vi "Autonomous Independent.vi"() -> ()   [LabVIEW 2016]
doc: "This VI is called when autonomous begins, and will automatically be terminated when autonomous ends. You can carry out timed or sensor driven robot movement independently without needing to return to the caller."
uses:
  <vilib>/Rock Robotics/Network Tables/NT Read Number.vi
  Global 2.vi
  Systems/Global 1.vi
panel:
  out "Elapsed Time (s) 2":dbl=0.2559828758239746 caption="Elapsed Time (s)"
  out "Time has Elapsed 2":bool=TRUE caption="Time has Elapsed"
  out "Present (s) 2":dbl=3576145380.999535 caption="Present (s)"
  out "Present (s)":dbl=3576102803.059525
  out "Time has Elapsed":bool=TRUE
  out "Elapsed Time (s)":dbl=0.25415611267089844
  out "Gyro":dbl=0.5670717799999513
  in  "Oscillate effort":dbl=0.25 format="%#_13g"
  out "Auto Mode":dbl=2.0
  in  "Auton_Modes":T1(array[cluster])=[{"Actions"=[{"Effort"=0.55, "Duration"=3.5, "Action"=enum."Nothing", "Encoder"=0.0, "Condition"=FALSE}, {"Effort"=0.0, "Duration"=0.0, "Action"=enum."Nothing", "Encoder"=0.0, "Condition"=FALSE}]}, {"Actions"=[{"Effort"=0.0, "Duration"=0.1, "Action"=enum."Drive Encoder Reset", "Encoder"=0.0, "Condition"=FALSE}, {"Effort"=0.0, "Duration"=0.1, "Action"=enum."Gyro Reset", "Encoder"=0.0, "Condition"=FALSE}, {"Effort"=0.0, "Duration"=4.0, "Action"=enum."Drive", "Encoder"=62.0, "Condition"=FALSE}, {"Effort"=0.15, "Duration"=0.1, "Action"=enum."Turn", "Encoder"=-55.0, "Condition"=FALSE}, {"Effort"=0.0, "Duration"=0.1, "Action"=enum."Gyro Reset", "Encoder"=0.0, "Condition"=FALSE}, {"Effort"=0.0, "Duration"=0.1, "Action"=enum."Drive Encoder Reset", "Encoder"=0.0, "Condition"=FALSE}, {"Effort"=0.0, "Duration"=4.0, "Action"=enum."Drive", "Encoder"=76.0, "Condition"=FALSE}, {"Effort"=1.0, "Duration"=0.25, "Action"=enum."Gear0", "Encoder"=0.0, "Condition"=FALSE}, {"Effort"=0.0, "Duration"=0.1, "Action"=enum."Drive Encoder Reset", "Encoder"=3.0, "Condition"=FALSE}, {"Effort"=0.0, "Duration"=3.0, "Action"=enum."Drive", "Encoder"=-36.0, "Condition"=FALSE}, {"Effort"=0.08, "Duration"=0.0, "Action"=enum."Turn", "Encoder"=15.5, "Condition"=FALSE}, {"Effort"=0.0, "Duration"=0.1, "Action"=enum."Gyro Reset", "Encoder"=0.0, "Condition"=FALSE}, {"Effort"=0.0, "Duration"=0.5, "Action"=enum."Drive Encoder Reset", "Encoder"=0.0, "Condition"=FALSE}, {"Effort"=0.0, "Duration"=5.0, "Action"=enum."Drive", "Encoder"=-94.0, "Condition"=TRUE}]}, {"Actions"=[{"Effort"=0.0, "Duration"=0.1, "Action"=enum."Drive Encoder Reset", "Encoder"=0.0, "Condition"=FALSE}, {"Effort"=0.0, "Duration"=0.1, "Action"=enum."Gyro Reset", "Encoder"=0.0, "Condition"=FALSE}, {"Effort"=0.11, "Duration"=4.0, "Action"=enum."Drive", "Encoder"=74.0, "Condition"=FALSE}, {"Effort"=1.0, "Duration"=0.5, "Action"=enum."Gear0", "Encoder"=0.0, "Condition"=FALSE}, {"Effort"=1.0, "Duration"=0.0, "Action"=enum."Nothing", "Encoder"=0.0, "Condition"=FALSE}, {"Effort"=1.0, "Duration"=0.0, "Action"=enum."Nothing", "Encoder"=0.0, "Condition"=FALSE}, {"Effort"=0.0, "Duration"=0.0, "Action"=enum."Drive Encoder Reset", "Encoder"=0.0, "Condition"=FALSE}, {"Effort"=0.0, "Duration"=0.0, "Action"=enum."Nothing", "Encoder"=0.0, "Condition"=FALSE}, {"Effort"=0.0, "Duration"=0.0, "Action"=enum."Nothing", "Encoder"=0.0, "Condition"=FALSE}, {"Effort"=0.0, "Duration"=10000.0, "Action"=enum."Drive", "Encoder"=-24.0, "Condition"=FALSE}, {"Effort"=0.0, "Duration"=0.0, "Action"=enum."Drive Encoder Reset", "Encoder"=0.0, "Condition"=FALSE}, {"Effort"=-0.4, "Duration"=5.0, "Action"=enum."Nothing", "Encoder"=70.0, "Condition"=FALSE}]}, {"Actions"=[{"Effort"=0.0, "Duration"=0.1, "Action"=enum."Drive Encoder Reset", "Encoder"=6.462, "Condition"=FALSE}, {"Effort"=0.0, "Duration"=0.1, "Action"=enum."Gyro Reset", "Encoder"=0.0, "Condition"=FALSE}, {"Effort"=0.0, "Duration"=1.0, "Action"=enum."Drive", "Encoder"=60.0, "Condition"=FALSE}, {"Effort"=0.15, "Duration"=0.1, "Action"=enum."Turn", "Encoder"=55.0, "Condition"=FALSE}, {"Effort"=0.0, "Duration"=0.1, "Action"=enum."Gyro Reset", "Encoder"=0.0, "Condition"=FALSE}, {"Effort"=-0.25, "Duration"=0.0, "Action"=enum."Drive Encoder Reset", "Encoder"=7.5, "Condition"=FALSE}, {"Effort"=0.0, "Duration"=4.0, "Action"=enum."Drive", "Encoder"=76.0, "Condition"=FALSE}, {"Effort"=1.0, "Duration"=0.25, "Action"=enum."Gear0", "Encoder"=0.0, "Condition"=FALSE}, {"Effort"=0.0, "Duration"=0.1, "Action"=enum."Drive Encoder Reset", "Encoder"=0.0, "Condition"=FALSE}, {"Effort"=0.0, "Duration"=3.0, "Action"=enum."Drive", "Encoder"=-36.0, "Condition"=FALSE}, {"Effort"=0.08, "Duration"=0.0, "Action"=enum."Turn", "Encoder"=-60.0, "Condition"=FALSE}, {"Effort"=0.0, "Duration"=0.1, "Action"=enum."Gyro Reset", "Encoder"=0.0, "Condition"=FALSE}, {"Effort"=0.0, "Duration"=0.5, "Action"=enum."Drive Encoder Reset", "Encoder"=0.0, "Condition"=FALSE}, {"Effort"=0.0, "Duration"=5.0, "Action"=enum."Drive", "Encoder"=30.0, "Condition"=TRUE}]}, {"Actions"=[{"Effort"=0.0, "Duration"=0.1, "Action"=enum."Drive Encoder Reset", "Encoder"=6.462, "Condition"=FALSE}, {"Effort"=0.0, "Duration"=0.1, "Action"=enum."Gyro Reset", "Encoder"=0.0, "Condition"=FALSE}, {"Effort"=0.0, "Duration"=1.0, "Action"=enum."Drive", "Encoder"=60.0, "Condition"=FALSE}, {"Effort"=0.15, "Duration"=0.1, "Action"=enum."Turn", "Encoder"=-55.0, "Condition"=FALSE}, {"Effort"=0.0, "Duration"=0.1, "Action"=enum."Gyro Reset", "Encoder"=0.0, "Condition"=FALSE}, {"Effort"=-0.25, "Duration"=0.0, "Action"=enum."Drive Encoder Reset", "Encoder"=7.5, "Condition"=FALSE}, {"Effort"=0.0, "Duration"=4.0, "Action"=enum."Drive", "Encoder"=76.0, "Condition"=FALSE}, {"Effort"=1.0, "Duration"=0.25, "Action"=enum."Gear0", "Encoder"=0.0, "Condition"=FALSE}, {"Effort"=0.0, "Duration"=0.1, "Action"=enum."Drive Encoder Reset", "Encoder"=0.0, "Condition"=FALSE}, {"Effort"=0.0, "Duration"=3.0, "Action"=enum."Drive", "Encoder"=-36.0, "Condition"=FALSE}, {"Effort"=0.08, "Duration"=0.0, "Action"=enum."Turn", "Encoder"=60.0, "Condition"=FALSE}, {"Effort"=0.0, "Duration"=0.1, "Action"=enum."Gyro Reset", "Encoder"=0.0, "Condition"=FALSE}, {"Effort"=0.0, "Duration"=0.5, "Action"=enum."Drive Encoder Reset", "Encoder"=0.0, "Condition"=FALSE}, {"Effort"=0.0, "Duration"=5.0, "Action"=enum."Drive", "Encoder"=30.0, "Condition"=TRUE}]}, {"Actions"=[{"Effort"=0.0, "Duration"=0.1, "Action"=enum."Drive Encoder Reset", "Encoder"=0.0, "Condition"=FALSE}, {"Effort"=0.0, "Duration"=0.1, "Action"=enum."Gyro Reset", "Encoder"=0.0, "Condition"=FALSE}, {"Effort"=0.0, "Duration"=4.0, "Action"=enum."Drive", "Encoder"=62.0, "Condition"=FALSE}, {"Effort"=0.15, "Duration"=0.1, "Action"=enum."Turn", "Encoder"=55.0, "Condition"=FALSE}, {"Effort"=0.0, "Duration"=0.1, "Action"=enum."Gyro Reset", "Encoder"=0.0, "Condition"=FALSE}, {"Effort"=0.0, "Duration"=0.1, "Action"=enum."Drive Encoder Reset", "Encoder"=0.0, "Condition"=FALSE}, {"Effort"=0.0, "Duration"=4.0, "Action"=enum."Drive", "Encoder"=76.0, "Condition"=FALSE}, {"Effort"=1.0, "Duration"=0.25, "Action"=enum."Gear0", "Encoder"=0.0, "Condition"=FALSE}, {"Effort"=0.0, "Duration"=0.1, "Action"=enum."Drive Encoder Reset", "Encoder"=3.0, "Condition"=FALSE}, {"Effort"=0.0, "Duration"=3.0, "Action"=enum."Drive", "Encoder"=-36.0, "Condition"=FALSE}, {"Effort"=0.08, "Duration"=0.0, "Action"=enum."Turn", "Encoder"=-15.5, "Condition"=FALSE}, {"Effort"=0.0, "Duration"=0.1, "Action"=enum."Gyro Reset", "Encoder"=0.0, "Condition"=FALSE}, {"Effort"=0.0, "Duration"=0.5, "Action"=enum."Drive Encoder Reset", "Encoder"=0.0, "Condition"=FALSE}, {"Effort"=0.0, "Duration"=5.0, "Action"=enum."Drive", "Encoder"=-94.0, "Condition"=TRUE}, {"Effort"=0.0, "Duration"=10.0, "Action"=enum."Shoot", "Encoder"=0.0, "Condition"=FALSE}]}, {"Actions"=[{"Effort"=0.0, "Duration"=0.1, "Action"=enum."Drive Encoder Reset", "Encoder"=0.0, "Condition"=FALSE}, {"Effort"=0.0, "Duration"=0.1, "Action"=enum."Gyro Reset", "Encoder"=0.0, "Condition"=FALSE}, {"Effort"=0.2, "Duration"=5.0, "Action"=enum."Drive", "Encoder"=110.0, "Condition"=FALSE}, {"Effort"=0.75, "Duration"=1.0, "Action"=enum."Nothing", "Encoder"=0.0, "Condition"=FALSE}, {"Effort"=0.0, "Duration"=1.0, "Action"=enum."Nothing", "Encoder"=0.0, "Condition"=FALSE}, {"Effort"=0.0, "Duration"=0.0, "Action"=enum."Nothing", "Encoder"=0.0, "Condition"=FALSE}]}, {"Actions"=[{"Effort"=0.0, "Duration"=0.1, "Action"=enum."Drive Encoder Reset", "Encoder"=0.0, "Condition"=FALSE}, {"Effort"=0.0, "Duration"=0.1, "Action"=enum."Gyro Reset", "Encoder"=0.0, "Condition"=FALSE}, {"Effort"=0.3, "Duration"=0.0, "Action"=enum."Drive", "Encoder"=24.0, "Condition"=FALSE}, {"Effort"=0.3, "Duration"=3.0, "Action"=enum."Nothing", "Encoder"=0.0, "Condition"=FALSE}, {"Effort"=0.3, "Duration"=2.0, "Action"=enum."Vision Correction", "Encoder"=30.0, "Condition"=FALSE}, {"Effort"=0.2, "Duration"=1.0, "Action"=enum."Drive", "Encoder"=18.5, "Condition"=TRUE}, {"Effort"=1.0, "Duration"=0.0, "Action"=enum."Gear0", "Encoder"=0.0, "Condition"=FALSE}, {"Effort"=-0.2, "Duration"=1.3, "Action"=enum."Drive", "Encoder"=30.0, "Condition"=TRUE}, {"Effort"=0.0, "Duration"=3.0, "Action"=enum."Nothing", "Encoder"=0.0, "Condition"=FALSE}, {"Effort"=0.03, "Duration"=0.0, "Action"=enum."Turn", "Encoder"=0.0, "Condition"=FALSE}, {"Effort"=0.0, "Duration"=0.0, "Action"=enum."Drive", "Encoder"=0.0, "Condition"=FALSE}]}, {"Actions"=[{"Effort"=0.0, "Duration"=0.0, "Action"=enum."Nothing", "Encoder"=0.0, "Condition"=FALSE}]}, {"Actions"=[{"Effort"=0.0, "Duration"=2.5, "Action"=enum."Shoot", "Encoder"=0.0, "Condition"=FALSE}, {"Effort"=0.0, "Duration"=5.0, "Action"=enum."Index", "Encoder"=0.0, "Condition"=FALSE}, {"Effort"=0.25, "Duration"=3.5, "Action"=enum."Nothing", "Encoder"=88.0, "Condition"=FALSE}, {"Effort"=1.0, "Duration"=1.0, "Action"=enum."Nothing", "Encoder"=0.0, "Condition"=FALSE}, {"Effort"=1.0, "Duration"=1.0, "Action"=enum."Nothing", "Encoder"=0.0, "Condition"=FALSE}, {"Effort"=1.0, "Duration"=0.5, "Action"=enum."Nothing", "Encoder"=0.0, "Condition"=FALSE}, {"Effort"=0.0, "Duration"=0.0, "Action"=enum."Nothing", "Encoder"=0.0, "Condition"=FALSE}, {"Effort"=-0.25, "Duration"=0.0, "Action"=enum."Nothing", "Encoder"=3.0, "Condition"=FALSE}, {"Effort"=0.0, "Duration"=0.0, "Action"=enum."Nothing", "Encoder"=0.0, "Condition"=FALSE}, {"Effort"=0.25, "Duration"=0.0, "Action"=enum."Nothing", "Encoder"=24.0, "Condition"=FALSE}, {"Effort"=0.0, "Duration"=0.0, "Action"=enum."Nothing", "Encoder"=0.0, "Condition"=FALSE}, {"Effort"=-0.25, "Duration"=0.0, "Action"=enum."Nothing", "Encoder"=12.0, "Condition"=FALSE}]}, {"Actions"=[{"Effort"=0.0, "Duration"=0.1, "Action"=enum."Drive Encoder Reset", "Encoder"=0.0, "Condition"=FALSE}, {"Effort"=0.0, "Duration"=1.0, "Action"=enum."Gyro Reset", "Encoder"=0.0, "Condition"=FALSE}, {"Effort"=0.3, "Duration"=1.4, "Action"=enum."Drive", "Encoder"=88.0, "Condition"=FALSE}, {"Effort"=0.3, "Duration"=3.0, "Action"=enum."Turn", "Encoder"=2.0, "Condition"=FALSE}, {"Effort"=1.0, "Duration"=1.0, "Action"=enum."Nothing", "Encoder"=0.0, "Condition"=FALSE}, {"Effort"=1.0, "Duration"=1.0, "Action"=enum."Nothing", "Encoder"=0.0, "Condition"=FALSE}, {"Effort"=0.0, "Duration"=0.0, "Action"=enum."Nothing", "Encoder"=0.0, "Condition"=FALSE}, {"Effort"=-0.25, "Duration"=0.0, "Action"=enum."Nothing", "Encoder"=3.0, "Condition"=FALSE}, {"Effort"=0.0, "Duration"=0.0, "Action"=enum."Nothing", "Encoder"=0.0, "Condition"=FALSE}, {"Effort"=0.25, "Duration"=0.0, "Action"=enum."Nothing", "Encoder"=24.0, "Condition"=FALSE}, {"Effort"=0.0, "Duration"=0.0, "Action"=enum."Nothing", "Encoder"=0.0, "Condition"=FALSE}, {"Effort"=-0.25, "Duration"=0.0, "Action"=enum."Nothing", "Encoder"=12.0, "Condition"=FALSE}]}, {"Actions"=[{"Effort"=0.0, "Duration"=1.0, "Action"=enum."Drive Encoder Reset", "Encoder"=0.0, "Condition"=FALSE}, {"Effort"=0.0, "Duration"=1.0, "Action"=enum."Shoot", "Encoder"=0.0, "Condition"=FALSE}, {"Effort"=0.25, "Duration"=5.0, "Action"=enum."Index", "Encoder"=88.0, "Condition"=FALSE}, {"Effort"=1.0, "Duration"=1.0, "Action"=enum."Nothing", "Encoder"=0.0, "Condition"=FALSE}, {"Effort"=1.0, "Duration"=1.0, "Action"=enum."Nothing", "Encoder"=0.0, "Condition"=FALSE}, {"Effort"=1.0, "Duration"=0.5, "Action"=enum."Nothing", "Encoder"=0.0, "Condition"=FALSE}, {"Effort"=0.0, "Duration"=0.0, "Action"=enum."Nothing", "Encoder"=0.0, "Condition"=FALSE}, {"Effort"=-0.25, "Duration"=0.0, "Action"=enum."Nothing", "Encoder"=3.0, "Condition"=FALSE}, {"Effort"=0.0, "Duration"=0.0, "Action"=enum."Nothing", "Encoder"=0.0, "Condition"=FALSE}, {"Effort"=0.25, "Duration"=0.0, "Action"=enum."Nothing", "Encoder"=24.0, "Condition"=FALSE}, {"Effort"=0.0, "Duration"=0.0, "Action"=enum."Nothing", "Encoder"=0.0, "Condition"=FALSE}, {"Effort"=-0.25, "Duration"=0.0, "Action"=enum."Nothing", "Encoder"=12.0, "Condition"=FALSE}]}, {"Actions"=[{"Effort"=0.0, "Duration"=0.1, "Action"=enum."Drive Encoder Reset", "Encoder"=0.0, "Condition"=FALSE}, {"Effort"=0.0, "Duration"=1.0, "Action"=enum."Gyro Reset", "Encoder"=0.0, "Condition"=FALSE}, {"Effort"=0.0, "Duration"=20.0, "Action"=enum."Drive", "Encoder"=60.0, "Condition"=FALSE}, {"Effort"=0.3, "Duration"=4.0, "Action"=enum."Nothing", "Encoder"=0.0, "Condition"=FALSE}, {"Effort"=1.0, "Duration"=1.0, "Action"=enum."Nothing", "Encoder"=0.0, "Condition"=FALSE}, {"Effort"=1.0, "Duration"=0.5, "Action"=enum."Nothing", "Encoder"=0.0, "Condition"=FALSE}, {"Effort"=0.0, "Duration"=0.0, "Action"=enum."Nothing", "Encoder"=0.0, "Condition"=FALSE}, {"Effort"=0.3, "Duration"=0.5, "Action"=enum."Nothing", "Encoder"=24.0, "Condition"=TRUE}, {"Effort"=0.0, "Duration"=0.0, "Action"=enum."Nothing", "Encoder"=0.0, "Condition"=FALSE}, {"Effort"=-0.2, "Duration"=2.0, "Action"=enum."Nothing", "Encoder"=24.0, "Condition"=TRUE}, {"Effort"=0.0, "Duration"=0.0, "Action"=enum."Nothing", "Encoder"=0.0, "Condition"=FALSE}, {"Effort"=-0.25, "Duration"=0.0, "Action"=enum."Nothing", "Encoder"=12.0, "Condition"=FALSE}]}, {"Actions"=[{"Effort"=0.0, "Duration"=0.1, "Action"=enum."Drive Encoder Reset", "Encoder"=0.0, "Condition"=FALSE}, {"Effort"=0.0, "Duration"=0.1, "Action"=enum."Gyro Reset", "Encoder"=0.0, "Condition"=FALSE}, {"Effort"=0.0, "Duration"=4.0, "Action"=enum."Nothing", "Encoder"=4.0, "Condition"=FALSE}, {"Effort"=0.3, "Duration"=0.1, "Action"=enum."Vision Correction", "Encoder"=24.0, "Condition"=FALSE}, {"Effort"=0.0, "Duration"=0.1, "Action"=enum."Nothing", "Encoder"=0.0, "Condition"=FALSE}, {"Effort"=0.3, "Duration"=4.0, "Action"=enum."Nothing", "Encoder"=68.17, "Condition"=FALSE}, {"Effort"=1.0, "Duration"=0.25, "Action"=enum."Nothing", "Encoder"=0.0, "Condition"=FALSE}, {"Effort"=0.0, "Duration"=0.0, "Action"=enum."Nothing", "Encoder"=3.0, "Condition"=FALSE}, {"Effort"=-0.3, "Duration"=3.0, "Action"=enum."Nothing", "Encoder"=36.0, "Condition"=FALSE}, {"Effort"=0.15, "Duration"=0.0, "Action"=enum."Nothing", "Encoder"=31.5, "Condition"=FALSE}, {"Effort"=0.0, "Duration"=0.1, "Action"=enum."Nothing", "Encoder"=0.0, "Condition"=FALSE}]}]
  # "Nothing"
  # "Boiler Right Right side gear"
  # "Middle Gear"
  # "Boiler Right Left Side Gear"
  # "Boiler Left RightSide Gear"
  # "Boiler Left Left Side Gear"
  # "Drive"
  # "Vision Correction"
  # "Hopper"
  # "10 ball"
  # "Farside"
  # "Boilerside-10 ball"
  # "Auto 5"
  # "Auto 6"
  # "Auto 6"
  # "Auto 7"
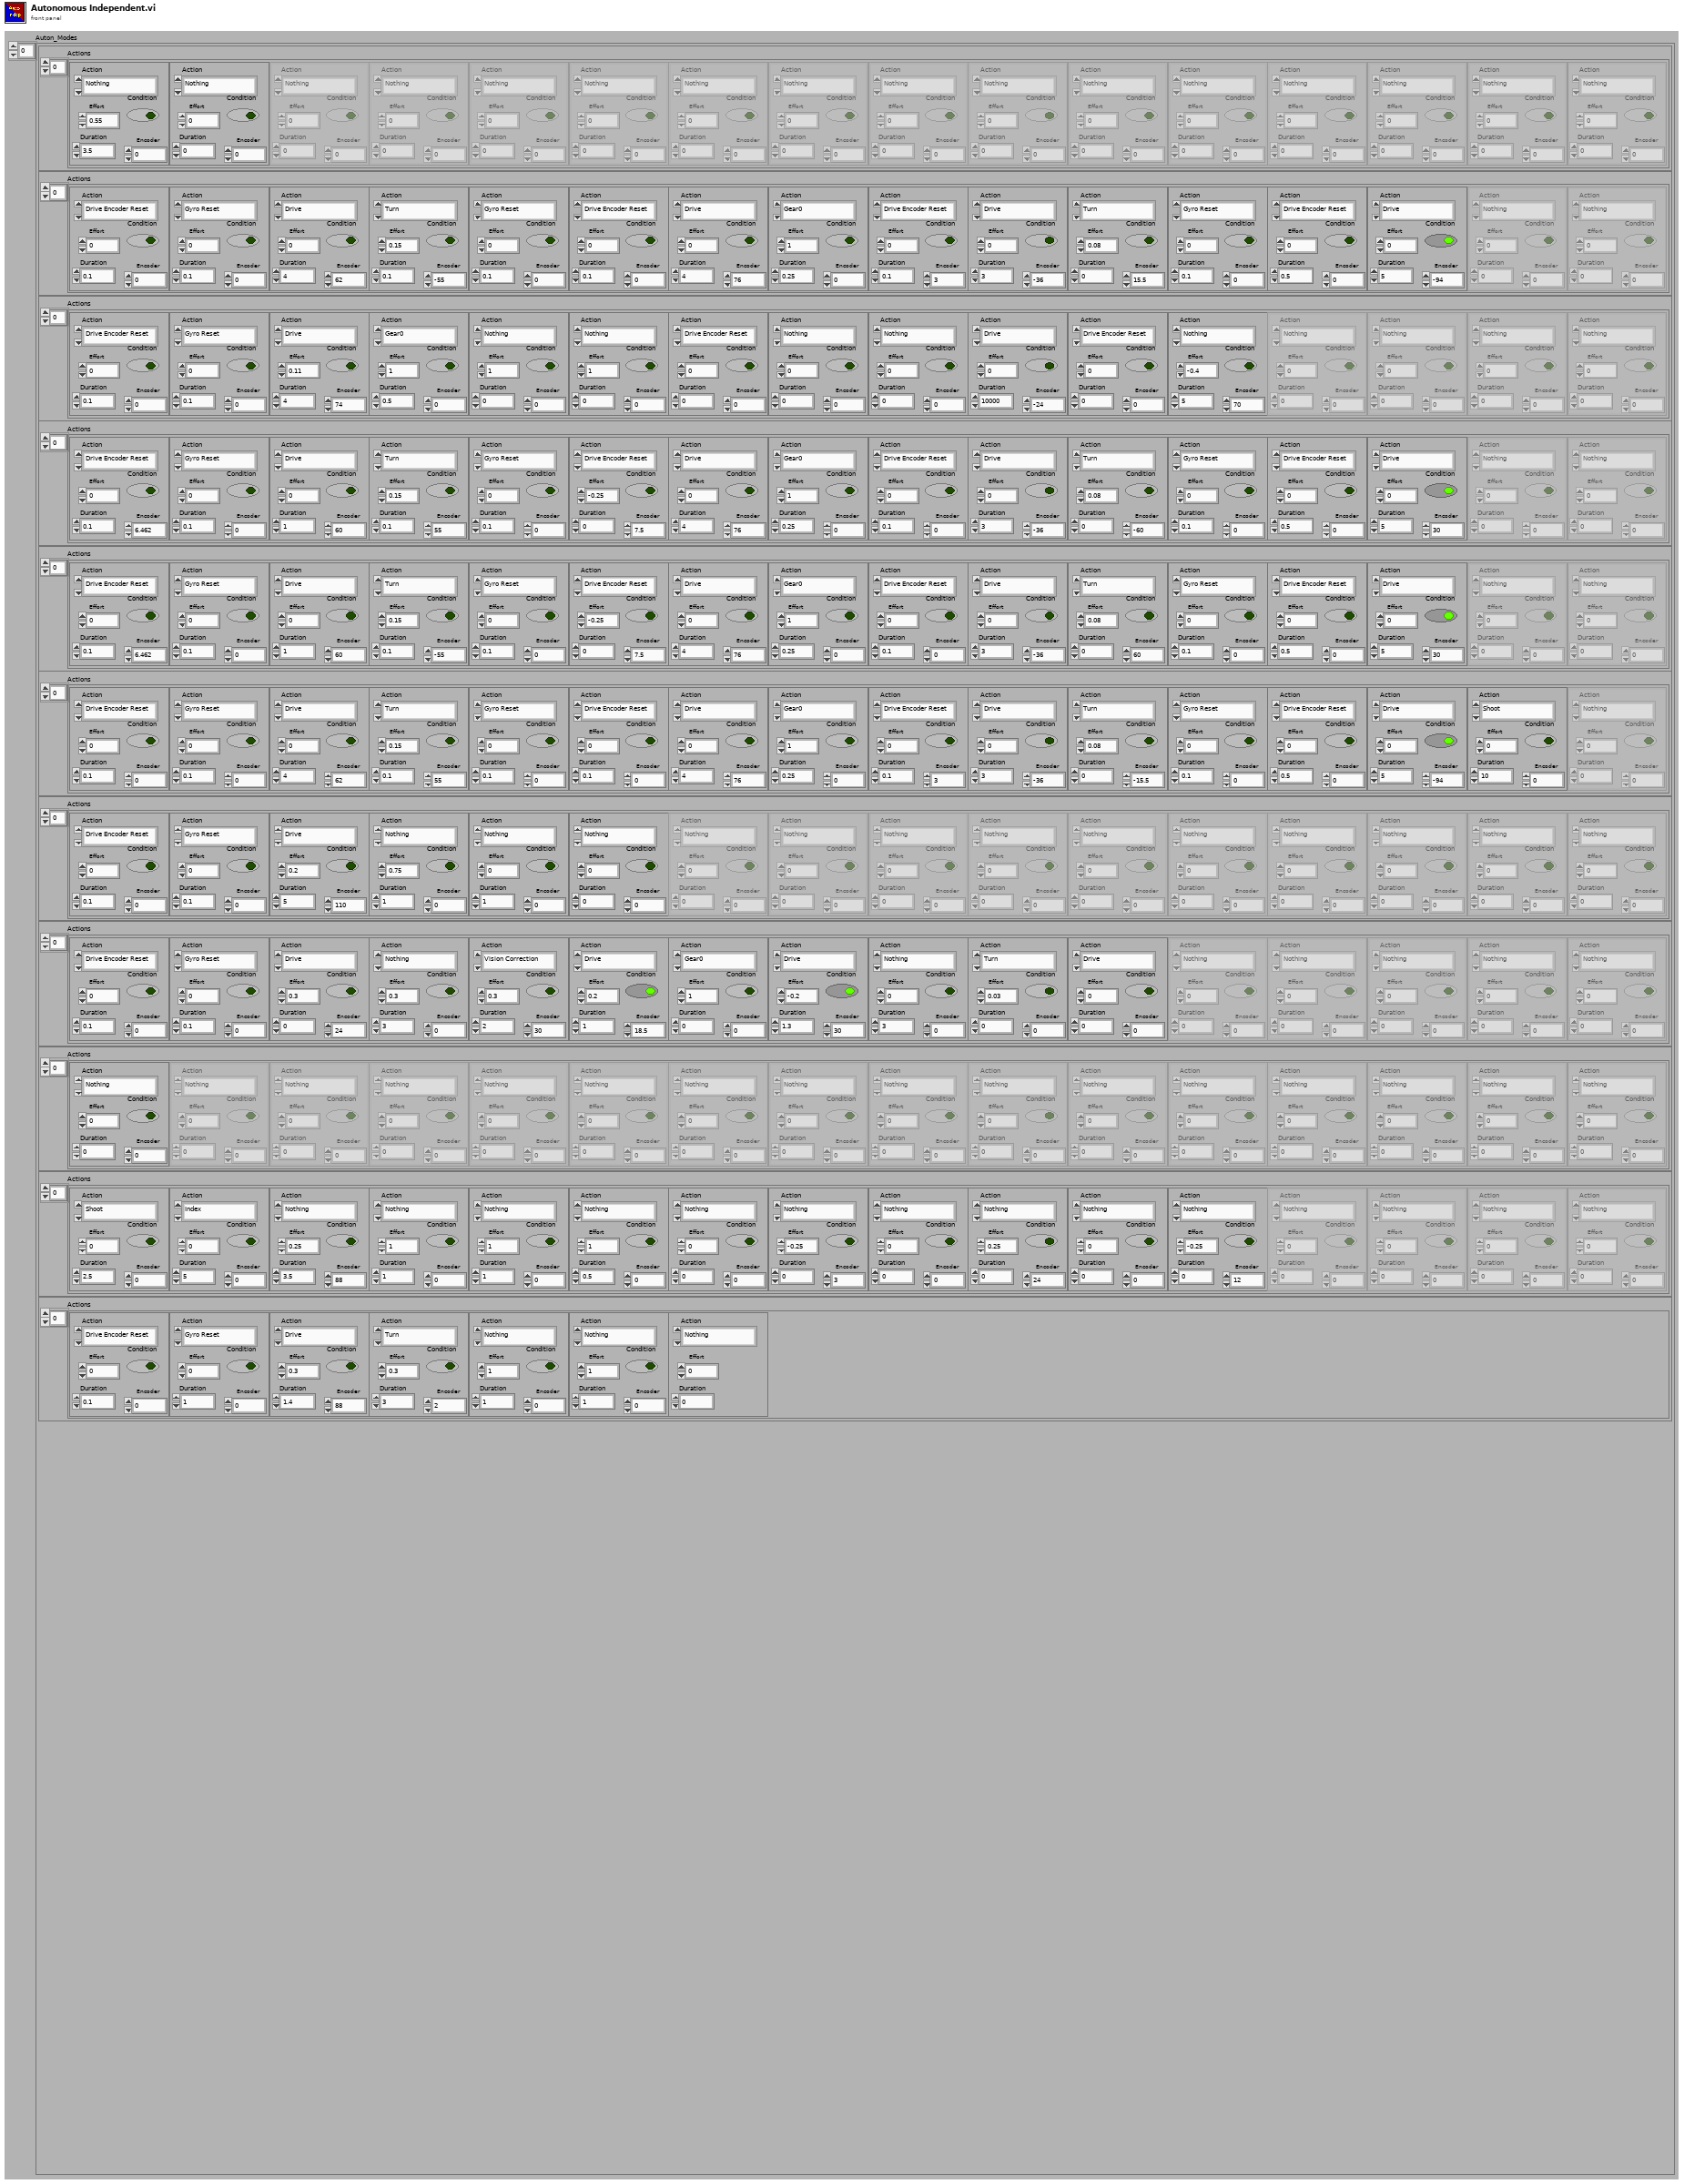
[diagram p1: front panel]
types:
  T1 = cluster{"Actions":cluster{"Effort":dbl, "Duration":dbl, "Action":enum16{"Nothing", "Drive", "Vision Correction", "Turn", "Gear0", "Gear1", "Climb", "Intake", "Index", "Shoot", "Test", "Drive Encoder Reset", "Gyro Reset"}, "Encoder":dbl, "Condition":bool}[]}[]
  T2 = cluster{"Actions":cluster{"Effort":dbl, "Duration":dbl, "Action":enum16{"Nothing", "Drive", "Vision Correction", "Turn", "Gear0", "Gear1", "Climb", "Intake", "Index", "Shoot", "Test", "Drive Encoder Reset", "Gyro Reset"}, "Encoder":dbl, "Condition":bool}[]}
  T3 = cluster{"Effort":dbl, "Duration":dbl, "Action":enum16{"Nothing", "Drive", "Vision Correction", "Turn", "Gear0", "Gear1", "Climb", "Intake", "Index", "Shoot", "Test", "Drive Encoder Reset", "Gyro Reset"}, "Encoder":dbl, "Condition":bool}[]
  T4 = enum16{"Nothing", "Drive", "Vision Correction", "Turn", "Gear0", "Gear1", "Climb", "Intake", "Index", "Shoot", "Test", "Drive Encoder Reset", "Gyro Reset"}
  T5 = typedef "WPI_MotorControlDeviceRef.ctl" = cluster{"DeviceStatus":errorcluster, "Type":T6, "PWM":cluster{"PWM Channel":T7, "DeadBand":T8}, "CAN":cluster{"Device Number":u8, "SetOutput VI Ref":variant, "GetOutput VI Ref":variant, "Enable VI Ref":variant, "Disable VI Ref":variant, "Data":variant}, "Invert":bool}
  T6 = typedef "WPI_MotorControlType.ctl" = enum16{"PWM", "CAN"}
  T7 = typedef "FPGA_DIOPWMChannel.ctl" = enum8{"PWM 0", "PWM 1", "PWM 2", "PWM 3", "PWM 4", "PWM 5", "PWM 6", "PWM 7", "PWM 8", "PWM 9", "PWM MXP 0", "PWM MXP 1", "PWM MXP 2", "PWM MXP 3", "PWM MXP 4", "PWM MXP 5", "PWM MXP 6", "PWM MXP 7", "PWM MXP 8", "PWM MXP 9", "Invalid"}
  T8 = typedef "WPI_PWMDeadband.ctl" = cluster{"Name":string, "maxPositivePwm":i32, "minPositivePwm":i32, "centerPwm":i32, "maxNegativePwm":i32, "minNegativePwm":i32, "angularRange":u16}
  T9 = typedef "WPI_CANTalonSRX_GlobalStatus.ctl" = cluster{"Applied Throttle":dbl, "Module Enabled":bool, "CAN Error":errorcluster, "Closed Loop Error":dbl, "Forward Limit Switch Closed":bool, "Reverse Limit Switch Closed":bool, "Sensor Position":dbl, "Sensor Velocity":dbl, "Current":dbl, "Sticky Fault - Over Temp":bool, "Sticky Fault - Under Voltage":bool, "Sticky Fault - Forward Limit":bool, "Sticky Fault - Reverse Limit":bool, "Sticky Fault - Forward Soft Limit":bool, "Sticky Fault - Reverse Soft Limit":bool, "Brake is Enabled":bool, "Encoder Position":dbl, "Encoder Velocity":dbl, "Encoder Index Count":dbl, "Encoder A Pin State":bool, "Encoder B Pin State":bool, "Encoder Index Pin State":bool, "Analog In":dbl, "Analog In Velocity":dbl, "Temperature (C)":dbl, "Battery Voltage":dbl, "Control 5 Is Supported":bool, "Current Profile Slot Select":dbl, "Pos Div 8":bool, "Vel Div 4":bool, "Pulse Width Position":i32, "Pulse Width Velocity":i32, "Pulse Width Rise To Rise (us)":i32, "Pulse Width Rise To Fall (us)":i32, "Mot Prof Active Is Under Run":bool, "Mot Prof Active Has Under Run":bool, "Mot Prof Active Is Last":bool, "Mot Prof Active Velocity Only":bool, "Mot Prof Active Is Valid":bool, "Mot Prof Buffer Is Full":bool, "Mot Prof Active Profile Slot Select":i32, "Mot Prof NextID":i32, "Mot Prof Count":i32, "Mot Prof Active Velocity":dbl, "Mot Prof Active Position":dbl, "Mot Prof Output Enable":i32}
  T10 = typedef "WPI_GyroDevRef.ctl" = cluster{"DevStatus":errorcluster, "Analog Channel":T11, "Offset":dbl, "Gain (VoltsPerDegree/Second)":dbl, "Gyro Type":enum16{"Analog", "XRS450"}, "Handle":i32, "SPI Bus":T12, "Device Found":bool, "Sample Rate":dbl, "Calibrate On Open":bool}
  T11 = typedef "FPGA_AIChannel.ctl" = enum8{"AI 0", "AI 1", "AI 2", "AI 3", "AI MXP 0", "AI MXP 1", "AI MXP 2", "AI MXP 3", "Invalid"}
  T12 = typedef "spi_bus.ctl" = enum16{"SPI On-Board, CS0", "SPI On-Board, CS1", "SPI On-Board, CS2", "SPI On-Board, CS3", "SPI MXP", "Invalid"}
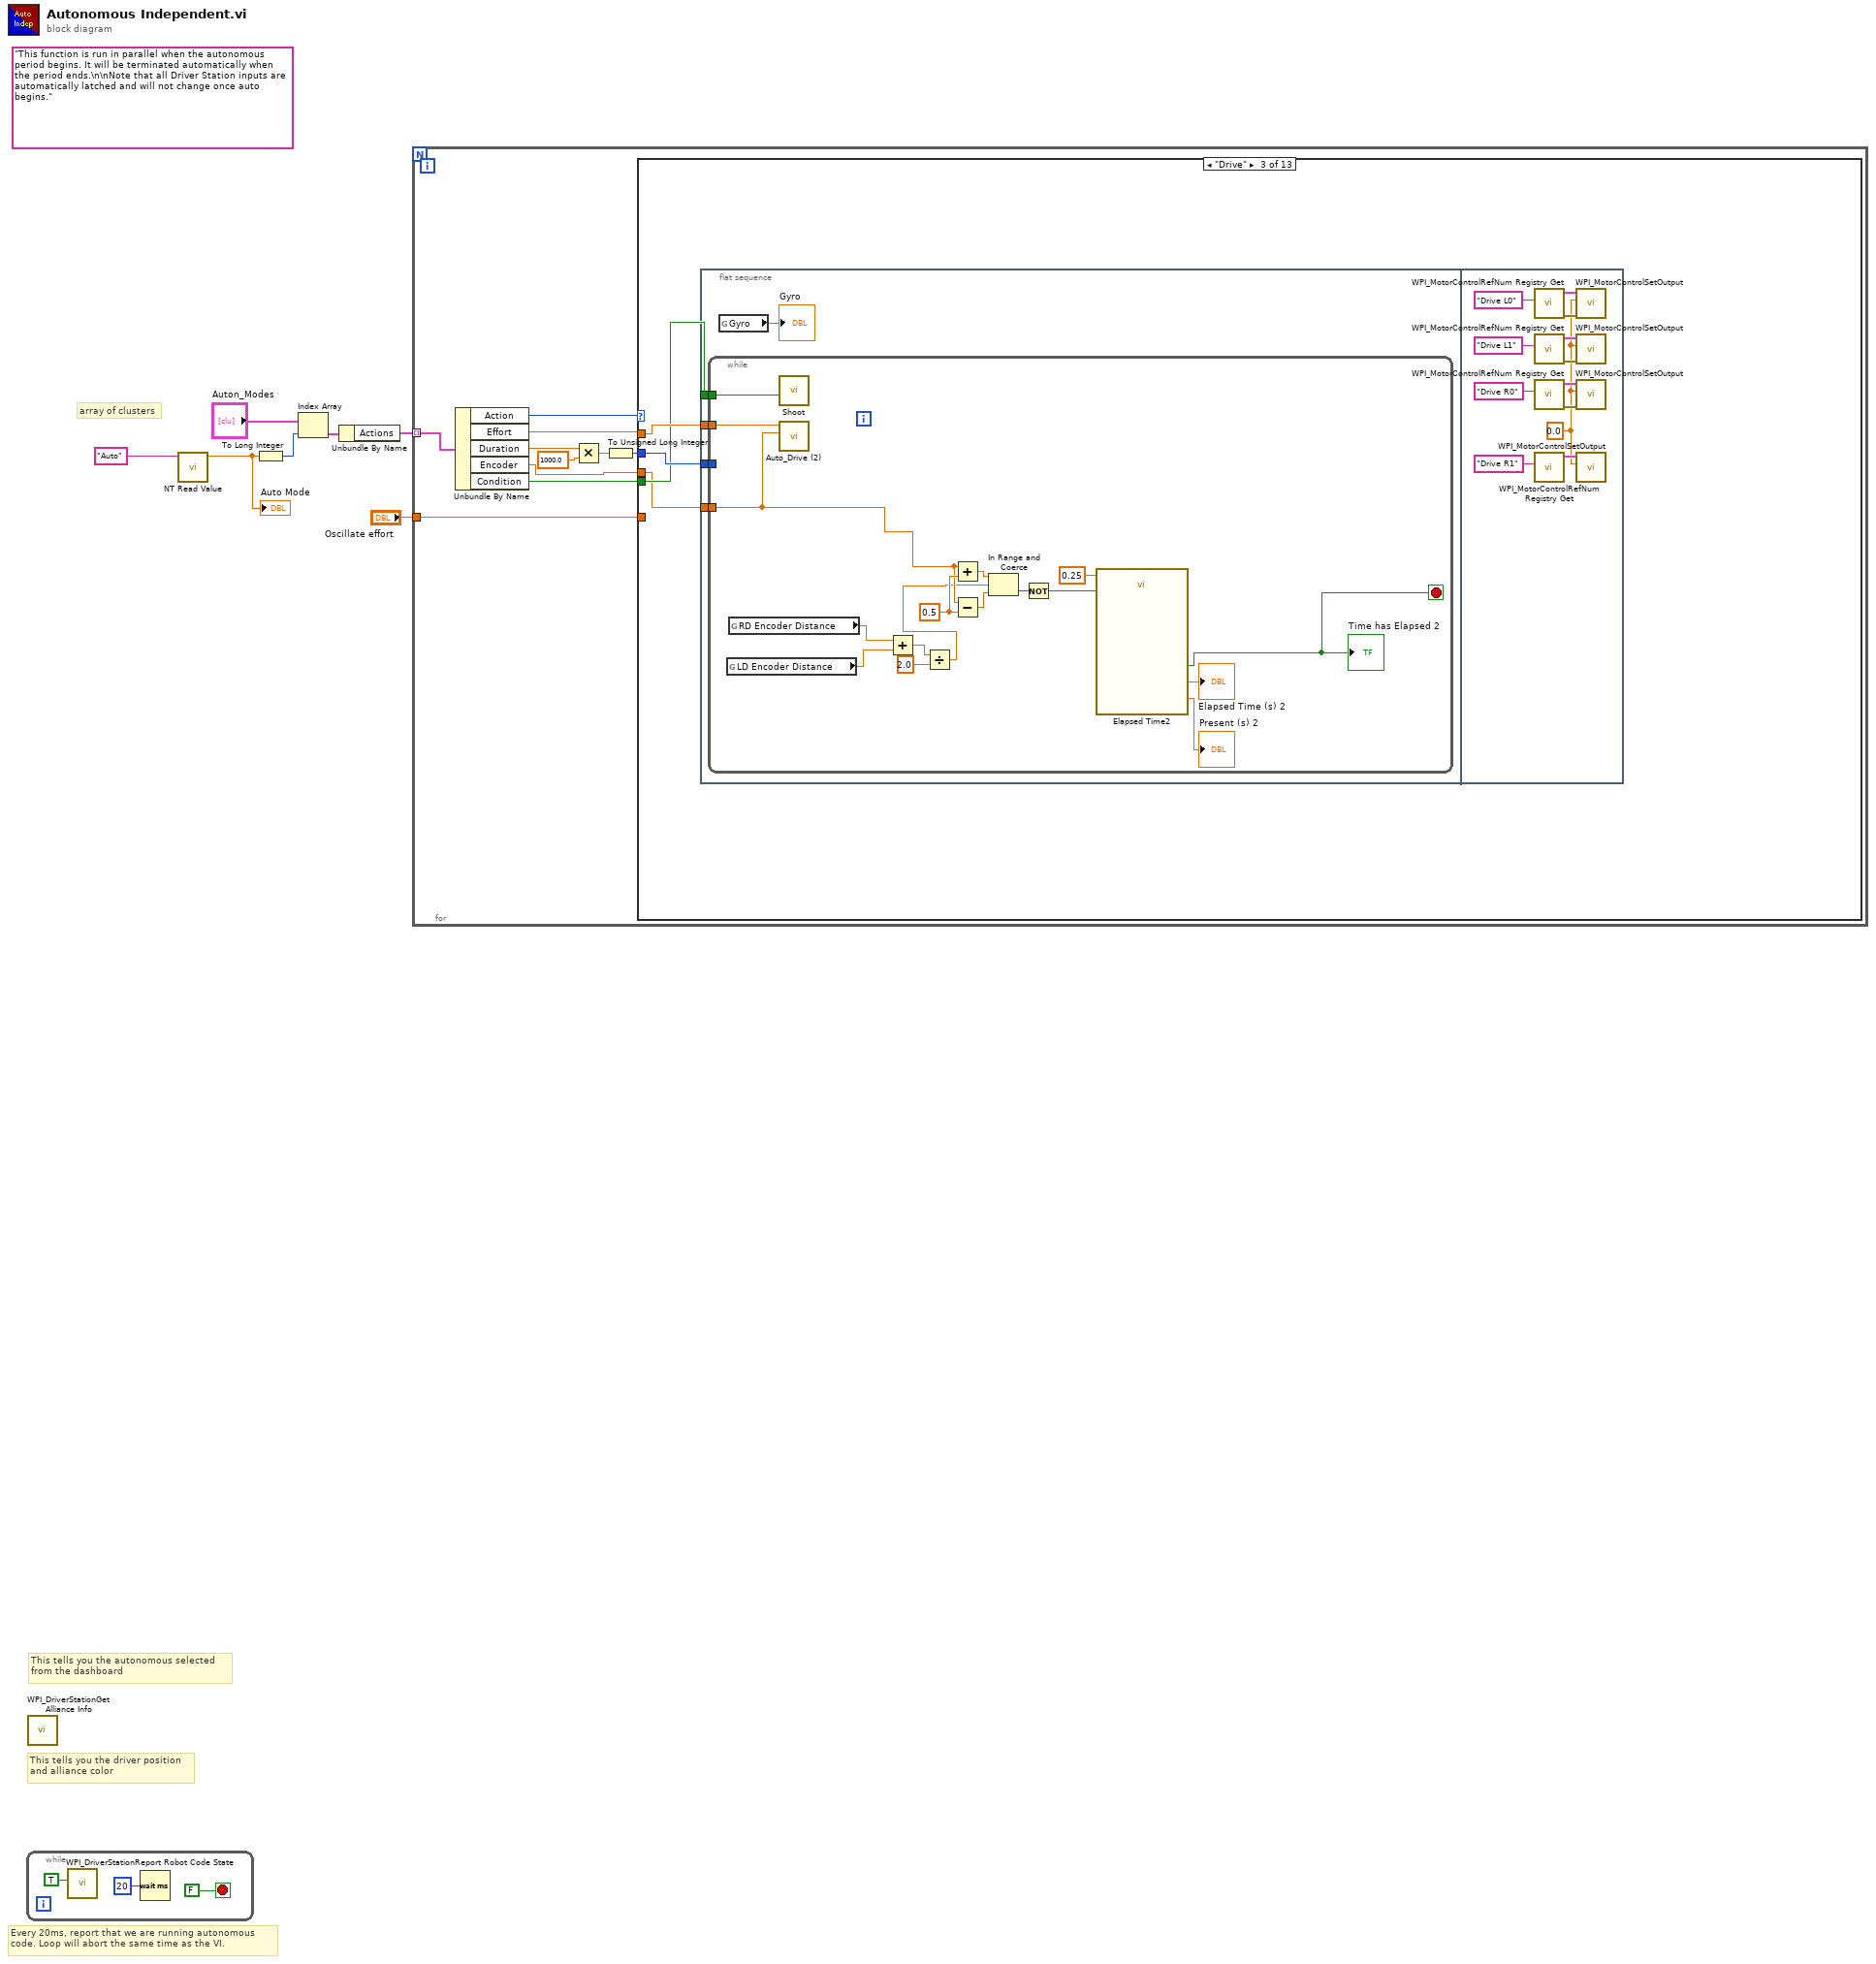
[diagram p0: block diagram]
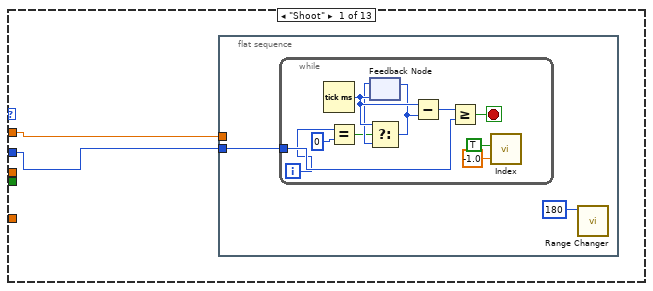
[diagram p2: hidden frame]
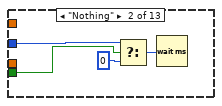
[diagram p3: hidden frame]
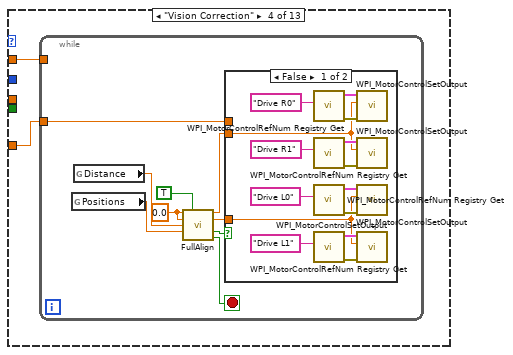
[diagram p4: hidden frame]
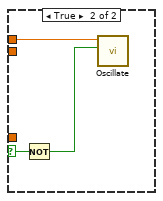
[diagram p5: hidden frame]
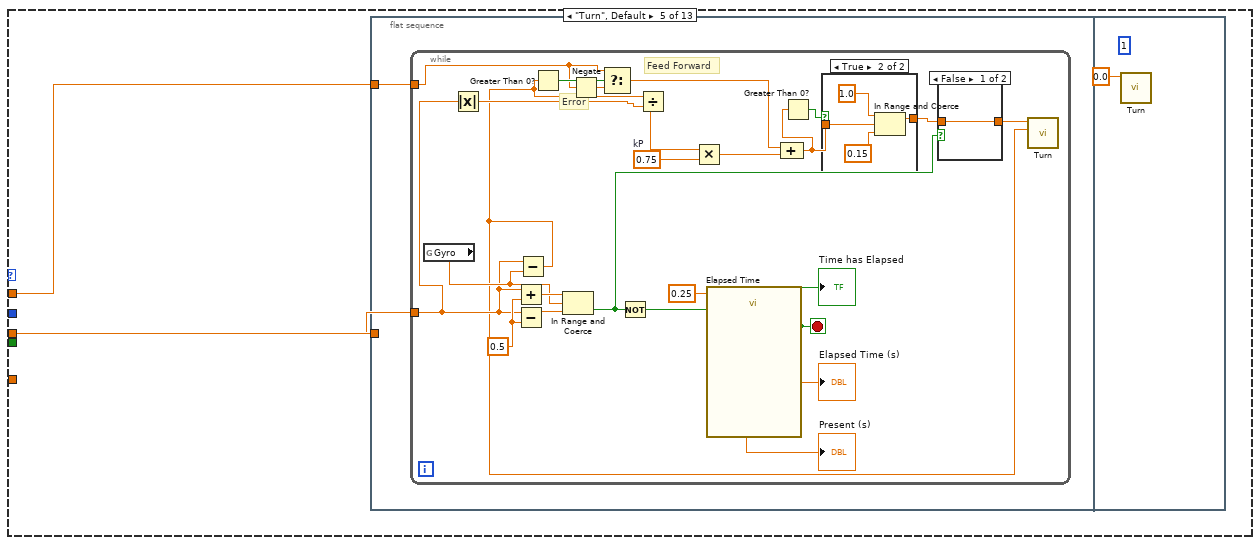
[diagram p6: hidden frame]
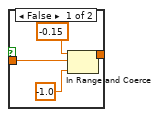
[diagram p7: hidden frame]
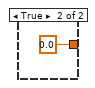
[diagram p8: hidden frame]
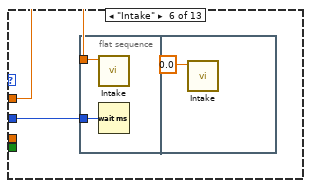
[diagram p9: hidden frame]
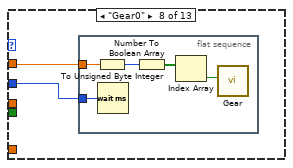
[diagram p11: hidden frame]
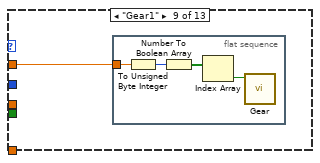
[diagram p12: hidden frame]
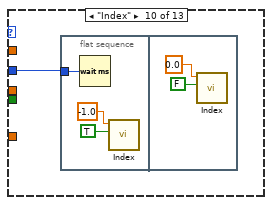
[diagram p13: hidden frame]
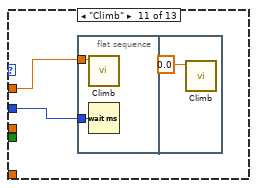
[diagram p14: hidden frame]
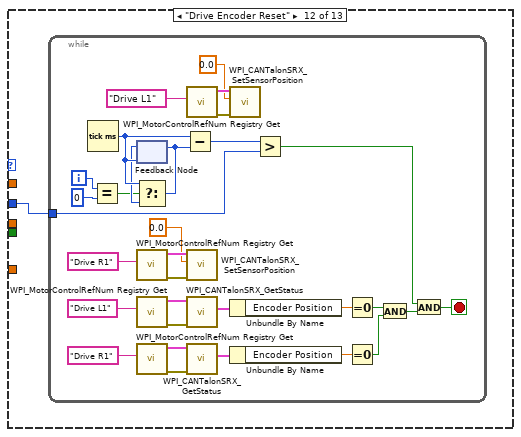
[diagram p15: hidden frame]
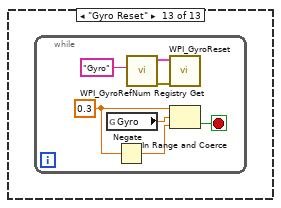
[diagram p16: hidden frame]
diagram:
  (unwired) "This function is run in parallel when the autonomous period begins. It will be terminated automatically when the period ends.\n\nNote that all Driver Station inputs are automatically latched and will not change once auto begins."
  # "This tells you the autonomous selected\nfrom the dashboard"
  # "array of clusters"
  # "Every 20ms, report that we are running autonomous\ncode. Loop will abort the same time as the VI."
  # "This tells you the driver position\nand alliance color"
  n1 = while {
    stop <- FALSE stop-if-true
    n2 = call <vilib>:"WPI_DriverStationReport Robot Code State.vi"("Autonomous"=TRUE) -> ()  [unwired: 10 in, 1 out]
    n3 = Wait (ms)(milliseconds to wait=u32 20) -> ()  [unwired: 1 out]
  }
  n4 = call <vilib>:"WPI_DriverStationGet Alliance Info.vi"() -> ()  [unwired: 12 out]
  n5 = call-poly <vilib>:"NT Read Value.vi"("Name"="Auto") -> ("Numeric"=w2:dbl)  [unwired: 9 in, 1 out]
  "Auto Mode" <- w2
  n6 = To Long Integer(number=w2) -> (32bit integer=w4:i32)
  n7 = Index Array(array="Auton_Modes", index=w4) -> (element=w6:T2)
  n8 = Unbundle By Name(w6) -> ("Actions"=w7:T3)
  n9 = for {
    tunnel: w7 -> [w20] mode=indexing
    tunnel: "Oscillate effort" -> [w12]
    n10 = Unbundle By Name(w20) -> ("Action"=w11:T4, "Effort"=w19:dbl, "Duration"=w18:dbl, "Encoder"=w13:dbl, "Condition"=w15:bool)
    n11 = Multiply(x=w18, y=1000.0) -> (x*y=w17:dbl)
    n12 = To Unsigned Long Integer(number=w17) -> (unsigned 32bit integer=w16:u32)
    n13 = case shown="\"Drive\"" w11 {
      tunnel: w19 -> [w22 _ w43 w79 w107 w146 _ w151 w157 _ w169 _ _]
      tunnel: w16 -> [w21 w38 w42 _ _ w145 _ w150 _ w162 w168 w173 _]
      tunnel: w15 -> [_ w39 w41 _ _ _ _ _ _ _ _ _ _]
      tunnel: w13 -> [_ _ w40 _ w106 _ _ _ _ _ _ _ _]
      tunnel: w12 -> [_ _ _ w78 _ _ _ _ _ _ _ _ _]
      frame "Shoot" {
        n14 = flat-sequence {
          tunnel: w22 -> [_]
          tunnel: w21 -> [w24]
          frame #0 {
            n15 = while {
              tunnel: w24 -> [w28]
              i -> [w27]
              stop <- w29 stop-if-true
              n16 = Tick Count (ms)() -> (millisecond timer value=w35:u32)
              n17 = Equal?(x=w27, y=0) -> (x = y?=w33:bool)
              n18 = feedback #1(w35) -> (w34:u32)
              n19 = Select(t=w35, s=w33, f=w34) -> (s? t:f=w31:u32)
              n20 = feedback-in #1(w31) -> ()
              n21 = Subtract(x=w35, y=w31) -> (x-y=w30:u32)
              n22 = Greater Or Equal?(x=w30, y=w28) -> (x >= y?=w29:bool)
              n23 = call "Index.vi"("Shoot"=TRUE, "Output"=-1.0) -> ()  [unwired: 10 in]
            }
            n24 = call "Range Changer.vi"("POV"=i16 180) -> ()  [unwired: 10 in, 1 out]
          }
        }
      }
      frame "Nothing" {
        n25 = Select(t=w38, s=w39, f=u32 0) -> (s? t:f=w36:u32)
        n26 = Wait (ms)(milliseconds to wait=w36) -> ()  [unwired: 1 out]
      }
      frame "Drive" {
        n27 = flat-sequence {
          tunnel: w43 -> [w48]
          tunnel: w42 -> [w44]
          tunnel: w41 -> [w46]
          tunnel: w40 -> [w47]
          frame #0 {
            n28 = while {
              tunnel: w48 -> [w65]
              tunnel: w47 -> [w55]
              tunnel: w46 -> [w64]
              tunnel: w44 -> [_]
              stop <- w49 stop-if-true
              w63 = 0.5
              n29 = global read "Global 2.vi" "LD Encoder Distance"() -> (w53:dbl)
              n30 = global read "Global 2.vi" "RD Encoder Distance"() -> (w54:dbl)
              n31 = call "Shoot.vi"("Shoot"=w64) -> ()  [unwired: 10 in]
              n32 = call "Auto_Drive (2).vi"("Target"=w55, "Drive Effort"=w65) -> ()  [unwired: 10 in]
              n33 = Add(x=w54, y=w53) -> (x+y=w52:dbl)
              n34 = Divide(x=w52, y=2.0) -> (x/y=w50:dbl)
              n35 = Add(x=w55, y=w63) -> (x+y=w62:dbl)
              n36 = Subtract(x=w55, y=w63) -> (x-y=w61:dbl)
              n37 = In Range and Coerce(upper limit=w62, x=w50, lower limit=w61) -> (In Range?=w56:bool)  [unwired: 1 out]
              n38 = Not(x=w56) -> (.not. x?=w57:bool)
              n39 = call "Elapsed Time2"("Time Target (s)"=0.25, "Reset"=w57) -> ("Present (s)"=→"Present (s) 2":dbl, "Elapsed Time (s)"=→"Elapsed Time (s) 2":dbl, "Time has Elapsed"=w49:bool)  [unwired: 10 in, 5 out]
              "Time has Elapsed 2" <- w49
            }
            n40 = global read "Global 2.vi" "Gyro"() -> (→"Gyro":dbl)
          }
          frame #1 {
            w66 = 0.0 ("Drive L")
            n41 = call <vilib>:"WPI_MotorControlRefNum Registry Get.vi"("refnum name"="Drive L0") -> ("error out"=w72:errorcluster, "MotorControlDevRef"=w73:T5)  [unwired: 9 in]
            n42 = call <vilib>:"WPI_MotorControlRefNum Registry Get.vi"("refnum name"="Drive L1") -> ("error out"=w76:errorcluster, "MotorControlDevRef"=w75:T5)  [unwired: 9 in]
            n43 = call <vilib>:"WPI_MotorControlRefNum Registry Get.vi"("refnum name"="Drive R0") -> ("error out"=w71:errorcluster, "MotorControlDevRef"=w67:T5)  [unwired: 9 in]
            n44 = call <vilib>:"WPI_MotorControlRefNum Registry Get.vi"("refnum name"="Drive R1") -> ("MotorControlDevRef"=w69:T5)  [unwired: 9 in, 1 out]
            n45 = call <vilib>:"WPI_MotorControlSetOutput.vi"("error in (no error)"=w72, "Output"=w66, "MotorControlDevRef"=w73) -> ()  [unwired: 6 in, 3 out]
            n46 = call <vilib>:"WPI_MotorControlSetOutput.vi"("error in (no error)"=w76, "Output"=w66, "MotorControlDevRef"=w75) -> ()  [unwired: 6 in, 3 out]
            n47 = call <vilib>:"WPI_MotorControlSetOutput.vi"("error in (no error)"=w71, "Output"=w66, "MotorControlDevRef"=w67) -> ()  [unwired: 6 in, 3 out]
            n48 = call <vilib>:"WPI_MotorControlSetOutput.vi"("Output"=w66, "MotorControlDevRef"=w69) -> ()  [unwired: 7 in, 3 out]
          }
        }
      }
      frame "Vision Correction" {
        n49 = while {
          tunnel: w79 -> [_]
          tunnel: w78 -> [w82]
          stop <- w83 stop-if-true
          w86 = 0.0
          n50 = global read "Global 1.vi" "Positions"() -> (w84:dbl)
          n51 = global read "Global 1.vi" "Distance"() -> (w85:dbl)
          n52 = call "FullAlign.vi"("Joystick 0"=w86, "Button"=TRUE, "Joystick 1"=w86, "Distance"=w85, "Angle"=w84) -> ("Right Motor"=w88:dbl, "Left Motor"=w87:dbl, "Not In Sight?"=w80:bool, "In Range?"=w83:bool)  [unwired: 7 in]
          n53 = case shown="False" w80 {
            selector: w80 -> [_ w104]
            tunnel: w88 -> [w90 _]
            tunnel: w87 -> [w89 _]
            tunnel: w82 -> [_ w105]
            frame False {
              n54 = call <vilib>:"WPI_MotorControlRefNum Registry Get.vi"("refnum name"="Drive R0") -> ("error out"=w96:errorcluster, "MotorControlDevRef"=w92:T5)  [unwired: 9 in]
              n55 = call <vilib>:"WPI_MotorControlRefNum Registry Get.vi"("refnum name"="Drive R1") -> ("error out"=w91:errorcluster, "MotorControlDevRef"=w94:T5)  [unwired: 9 in]
              n56 = call <vilib>:"WPI_MotorControlRefNum Registry Get.vi"("refnum name"="Drive L0") -> ("error out"=w97:errorcluster, "MotorControlDevRef"=w98:T5)  [unwired: 9 in]
              n57 = call <vilib>:"WPI_MotorControlRefNum Registry Get.vi"("refnum name"="Drive L1") -> ("error out"=w101:errorcluster, "MotorControlDevRef"=w100:T5)  [unwired: 9 in]
              n58 = call <vilib>:"WPI_MotorControlSetOutput.vi"("error in (no error)"=w96, "Output"=w90, "MotorControlDevRef"=w92) -> ()  [unwired: 6 in, 3 out]
              n59 = call <vilib>:"WPI_MotorControlSetOutput.vi"("error in (no error)"=w91, "Output"=w90, "MotorControlDevRef"=w94) -> ()  [unwired: 6 in, 3 out]
              n60 = call <vilib>:"WPI_MotorControlSetOutput.vi"("error in (no error)"=w97, "Output"=w89, "MotorControlDevRef"=w98) -> ()  [unwired: 6 in, 3 out]
              n61 = call <vilib>:"WPI_MotorControlSetOutput.vi"("error in (no error)"=w101, "Output"=w89, "MotorControlDevRef"=w100) -> ()  [unwired: 6 in, 3 out]
            }
            frame True {
              n62 = Not(x=w104) -> (.not. x?=w103:bool)
              n63 = call "Oscillate.vi"("Target In Sight?"=w103, "Effort"=w105) -> ()  [unwired: 10 in]
            }
          }
        }
      }
      frame "Turn", Default {
        n64 = flat-sequence {
          tunnel: w107 -> [w109]
          tunnel: w106 -> [w108]
          frame #0 {
            n65 = while {
              tunnel: w109 -> [w114]
              tunnel: w108 -> [w119]
              stop <- w126 stop-if-true
              w122 = 0.75  # kP
              w133 = 0.5
              # "Feed Forward"
              # "Error"
              n66 = global read "Global 2.vi" "Gyro"() -> (w123:dbl)
              n67 = Absolute Value(x=w119) -> (abs(x)=w118:dbl)
              n68 = Add(x=w119, y=w133) -> (x+y=w132:dbl)
              n69 = Subtract(x=w119, y=w133) -> (x-y=w131:dbl)
              n70 = Subtract(x=w119, y=w123) -> (x-y=w115:dbl)
              n71 = Greater Than 0?(x=w115) -> (x > 0?=w117:bool)
              n72 = In Range and Coerce(upper limit=w132, x=w123, lower limit=w131) -> (In Range?=w125:bool)  [unwired: 1 out]
              n73 = Negate(x=w114) -> (-x=w116:dbl)
              n74 = Select(t=w114, s=w117, f=w116) -> (s? t:f=w113:dbl)
              n75 = Not(x=w125) -> (.not. x?=w127:bool)
              n76 = Divide(x=w115, y=w118) -> (x/y=w120:dbl)
              n77 = Multiply(x=w120, y=w122) -> (x*y=w121:dbl)
              n78 = call "Elapsed Time"("Time Target (s)"=0.25, "Reset"=w127) -> ("Present (s)"=→"Present (s)":dbl, "Elapsed Time (s)"=→"Elapsed Time (s)":dbl, "Time has Elapsed"=w126:bool)  [unwired: 10 in, 5 out]
              "Time has Elapsed" <- w126
              n79 = Compound Arithmetic op=ADD(w113, w121) -> (w110:dbl)
              n80 = Greater Than 0?(x=w110) -> (x > 0?=w111:bool)
              n81 = case shown="True" w111 {
                tunnel: [w134 w139] -> w112
                tunnel: w110 -> [w135 w138]
                frame False {
                  n82 = In Range and Coerce(upper limit=-0.15, x=w135, lower limit=-1.0) -> (coerced(x)=w134:dbl)  [unwired: 1 out]
                }
                frame True {
                  n83 = In Range and Coerce(upper limit=1.0, x=w138, lower limit=0.15) -> (coerced(x)=w139:dbl)  [unwired: 1 out]
                }
              }
              n84 = case shown="False" w125 {
                tunnel: [w142 0.0] -> w124
                tunnel: w112 -> [w142 _]
                frame False {
                }
                frame True {
                }
              }
              n85 = call "Turn.vi"("Gyro"=w115, "Effort"=w124) -> ()  [unwired: 10 in]
            }
          }
          frame #1 {
            (unwired) 1 ("mode")
            n86 = call "Turn.vi"("Effort"=0.0) -> ()  [unwired: 11 in]
          }
        }
      }
      frame "Intake" {
        n87 = flat-sequence {
          tunnel: w146 -> [w148]
          tunnel: w145 -> [w147]
          frame #0 {
            n88 = call "Intake.vi"("Effort"=w148) -> ()  [unwired: 11 in]
            n89 = Wait (ms)(milliseconds to wait=w147) -> ()  [unwired: 1 out]
          }
          frame #1 {
            n90 = call "Intake.vi"("Effort"=0.0) -> ()  [unwired: 11 in]
          }
        }
      }
      frame "Test" {
      }
      frame "Gear0" {
        n91 = flat-sequence {
          tunnel: w151 -> [w156]
          tunnel: w150 -> [w152]
          frame #0 {
            n92 = To Unsigned Byte Integer(number=w156) -> (unsigned 8bit integer=w155:u8)
            n93 = Wait (ms)(milliseconds to wait=w152) -> ()  [unwired: 1 out]
            n94 = Number To Boolean Array(number=w155) -> (Boolean array=w154:bool[])
            n95 = Index Array(array=w154) -> (element=w153:bool)  [unwired: 1 in]
            n96 = call "Gear.vi"("Gear0?"=w153) -> ()  [unwired: 11 in]
          }
        }
      }
      frame "Gear1" {
        n97 = flat-sequence {
          tunnel: w157 -> [w161]
          frame #0 {
            n98 = To Unsigned Byte Integer(number=w161) -> (unsigned 8bit integer=w160:u8)
            n99 = Number To Boolean Array(number=w160) -> (Boolean array=w159:bool[])
            n100 = Index Array(array=w159) -> (element=w158:bool)  [unwired: 1 in]
            n101 = call "Gear.vi"("Gear1?"=w158) -> ()  [unwired: 11 in]
          }
        }
      }
      frame "Index" {
        n102 = flat-sequence {
          tunnel: w162 -> [w163]
          frame #0 {
            n103 = Wait (ms)(milliseconds to wait=w163) -> ()  [unwired: 1 out]
            n104 = call "Index.vi"("Shoot"=TRUE ("Override?"), "Output"=-1.0) -> ()  [unwired: 10 in]
          }
          frame #1 {
            n105 = call "Index.vi"("Shoot"=FALSE ("Override?"), "Output"=0.0) -> ()  [unwired: 10 in]
          }
        }
      }
      frame "Climb" {
        n106 = flat-sequence {
          tunnel: w169 -> [w171]
          tunnel: w168 -> [w170]
          frame #0 {
            n107 = call "Climb.vi"("Effort"=w171) -> ()  [unwired: 11 in]
            n108 = Wait (ms)(milliseconds to wait=w170) -> ()  [unwired: 1 out]
          }
          frame #1 {
            n109 = call "Climb.vi"("Effort"=0.0) -> ()  [unwired: 11 in]
          }
        }
      }
      frame "Drive Encoder Reset" {
        n110 = while {
          tunnel: w173 -> [w176]
          i -> [w178]
          stop <- w174 stop-if-true
          n111 = Tick Count (ms)() -> (millisecond timer value=w184:u32)
          n112 = Equal?(x=w178, y=0) -> (x = y?=w182:bool)
          n113 = feedback #2(w184) -> (w183:u32)
          n114 = Select(t=w184, s=w182, f=w183) -> (s? t:f=w180:u32)
          n115 = feedback-in #2(w180) -> ()
          n116 = call <vilib>:"WPI_MotorControlRefNum Registry Get.vi"("refnum name"="Drive R1") -> ("error out"=w199:errorcluster, "MotorControlDevRef"=w198:T5)  [unwired: 9 in]
          n117 = call <vilib>:"WPI_MotorControlRefNum Registry Get.vi"("refnum name"="Drive L1") -> ("error out"=w194:errorcluster, "MotorControlDevRef"=w189:T5)  [unwired: 9 in]
          n118 = call <vilib>:"WPI_MotorControlRefNum Registry Get.vi"("refnum name"="Drive R1") -> ("error out"=w191:errorcluster, "MotorControlDevRef"=w190:T5)  [unwired: 9 in]
          n119 = Subtract(x=w184, y=w180) -> (x-y=w177:u32)
          n120 = call <vilib>:"WPI_MotorControlRefNum Registry Get.vi"("refnum name"="Drive L1") -> ("error out"=w201:errorcluster, "MotorControlDevRef"=w202:T5)  [unwired: 9 in]
          n121 = call <vilib>:"WPI_CANTalonSRX_SetSensorPosition.vi"("error in (no error)"=w199, "New Sensor Position"=0.0, "CAN Talon SRX Ref"=w198) -> ()  [unwired: 7 in, 2 out]
          n122 = call <vilib>:"WPI_CANTalonSRX_GetStatus.vi"("error in (no error)"=w194, "CAN Talon SRX Ref"=w189) -> ("Talon SRX Status"=w192:T9)  [unwired: 7 in, 2 out]
          n123 = call <vilib>:"WPI_CANTalonSRX_GetStatus.vi"("error in (no error)"=w191, "CAN Talon SRX Ref"=w190) -> ("Talon SRX Status"=w193:T9)  [unwired: 7 in, 2 out]
          n124 = call <vilib>:"WPI_CANTalonSRX_SetSensorPosition.vi"("error in (no error)"=w201, "New Sensor Position"=0.0, "CAN Talon SRX Ref"=w202) -> ()  [unwired: 7 in, 2 out]
          n125 = Unbundle By Name(w192) -> ("Encoder Position"=w187:dbl)
          n126 = Unbundle By Name(w193) -> ("Encoder Position"=w188:dbl)
          n127 = Greater?(x=w177, y=w176) -> (0:w175:bool)
          n128 = Equal To 0?(x=w187) -> (x = 0?=w186:bool)
          n129 = Equal To 0?(x=w188) -> (x = 0?=w185:bool)
          n130 = And(x=w186, y=w185) -> (x .and. y?=w179:bool)
          n131 = And(x=w175, y=w179) -> (x .and. y?=w174:bool)
        }
      }
      frame "Gyro Reset" {
        n132 = while {
          stop <- w205 stop-if-true
          w208 = 0.3
          n133 = global read "Global 2.vi" "Gyro"() -> (w206:dbl)
          n134 = Negate(x=w208) -> (-x=w207:dbl)
          n135 = call <vilib>:"WPI_GyroRefNum Registry Get.vi"("refnum name"="Gyro") -> ("error out"=w210:errorcluster, "GyroDevRef"=w211:T10)  [unwired: 9 in]
          n136 = call <vilib>:"WPI_GyroReset.vi"("error in"=w210, "GyroDevRef"=w211) -> ()  [unwired: 8 in, 2 out]
          n137 = In Range and Coerce(upper limit=w208, x=w206, lower limit=w207) -> (In Range?=w205:bool)  [unwired: 1 out]
        }
      }
    }
  }
